vi "TCP - Engine.vi"() -> ()   [LabVIEW 2017]
uses:
  TCP Host/Controls/Read File.ctl
  Controls/RT- Queue States.ctl
  Controls/TCP - Test Settings.ctl
  Controls/TCP - Signal Names.ctl
  Controls/TCP - Signals.ctl
  Controls/TCP - Driver control.ctl
  Variable/SubVI - Global.vi
panel:
  out "Waveform Chart":u32(graph)
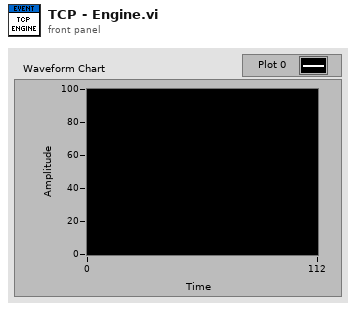
[diagram p1: front panel]
types:
  T1 = typedef "RT- Queue States.ctl" = enum16{"Initialize", "Enqueue", "Enqueue Priority", "Dequeue", "Flush", "Destroy"}
  T2 = typedef "Read File.ctl" = enum16{"Fetch XML", "Open", "Read", "Write", "Close"}
  T3 = typedef "TCP - Driver control.ctl" = enum16{"Init", "Load Sequence File", "Test Running", "Index Step", "Execute Step", "Send Results", "Sequence Complete", "Sequence Aborted", "Stop Sequence Triggered", "Update Manual Values", "Start Aux Logging", "Stop Aux Logging", "Change Dyno Selection", "Reset Emergency Fault", "Get Dyno Config", "Exit"}
  T4 = typedef "TCP - Test Settings.ctl" = cluster{"Sequence File":string, "Iteration":i32}
  T5 = typedef "TCP - Signals.ctl" = cluster{"Signal":T6, "Value":bool, "Data":variant}
  T6 = typedef "TCP - Signal Names.ctl" = enum16{"Test Running", "Start Test", "Test Started", "Sequence Complete", "Seuence Aborted", "Abort Test", "Test Settings Updated", "Log Path", "Update Manual Values", "Start Aux Logging", "Aux Log Started", "Stop Aux Logging", "Aux Log Stopped", "Set Dyno Config", "Get PID Values", "Reset Emergency", "Copy Log File", "Download Files", "Send Test Details", "Generate Alarm"}
  T7 = cluster{"Test details":cluster{"Furnace":string, "Material":string, "Angle":string, "ID":string, "Flowrate":string, "Test Name":string, "Tested By":string}, "Datalog Duration":dbl}
  T8 = cluster{"Furnace":string, "Material":string, "Angle":string, "ID":string, "Flowrate":string, "Test Name":string, "Tested By":string}
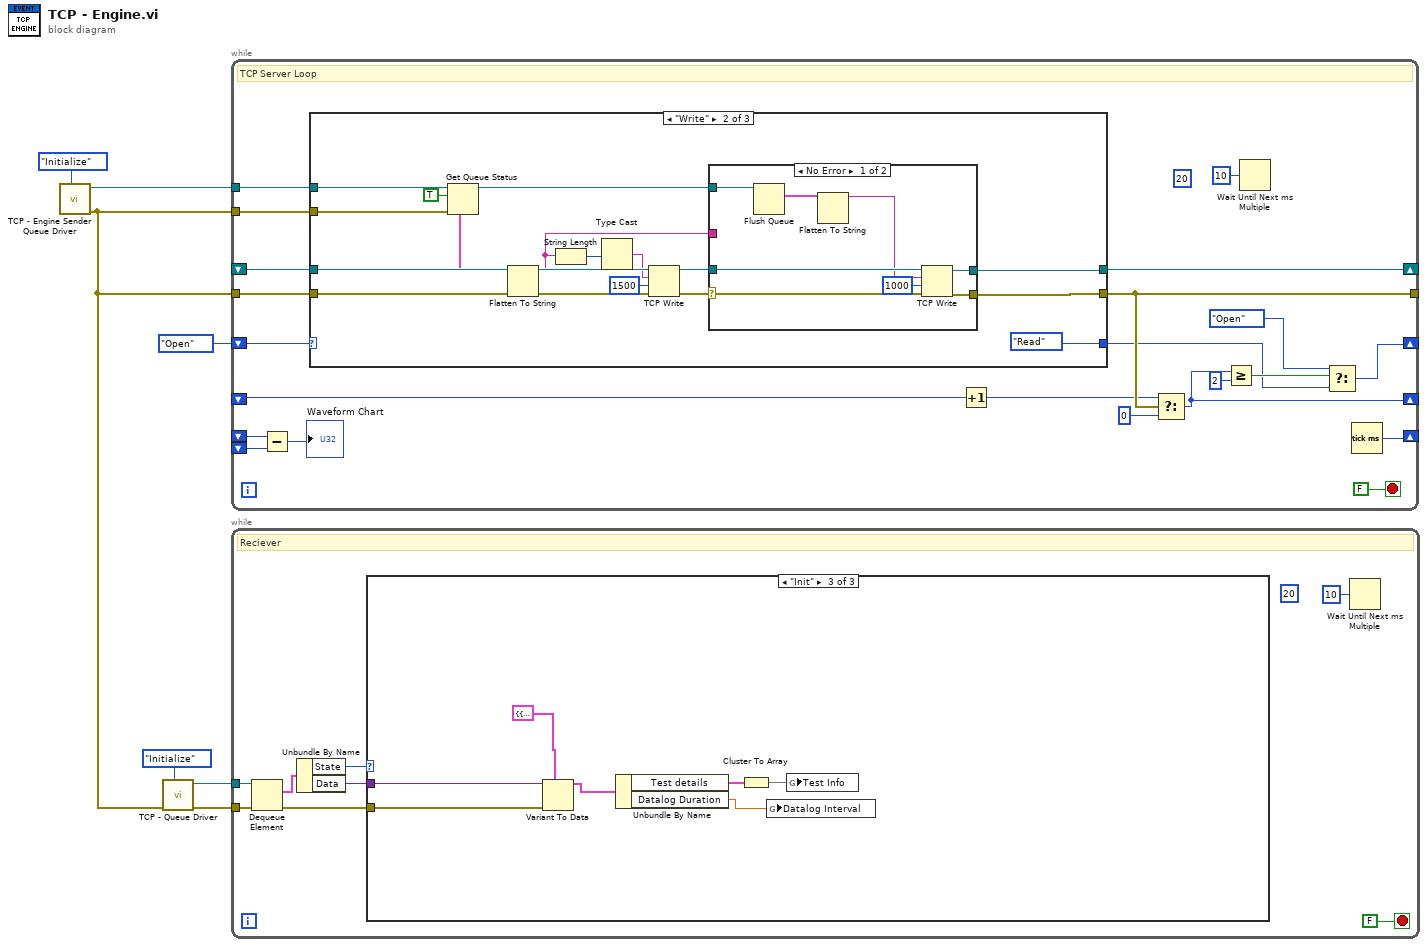
[diagram p0: block diagram]
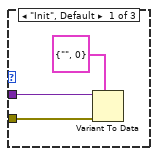
[diagram p2: hidden frame]
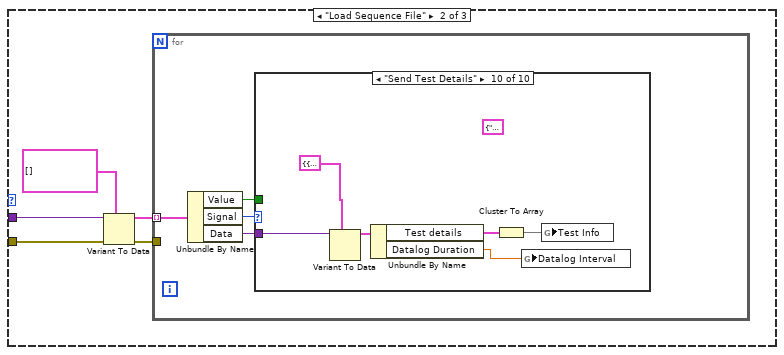
[diagram p3: hidden frame]
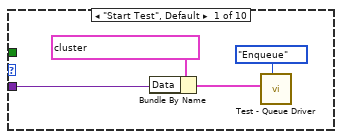
[diagram p4: hidden frame]
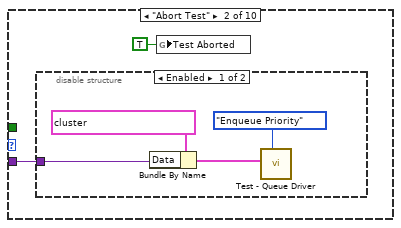
[diagram p5: hidden frame]
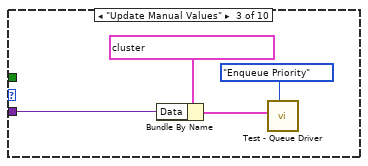
[diagram p7: hidden frame]
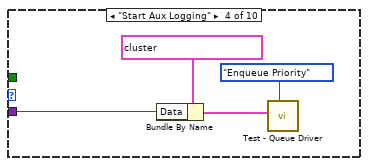
[diagram p8: hidden frame]
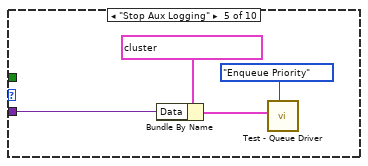
[diagram p9: hidden frame]
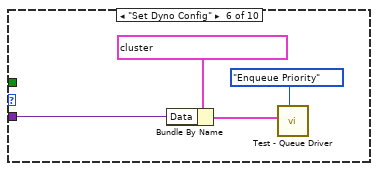
[diagram p10: hidden frame]
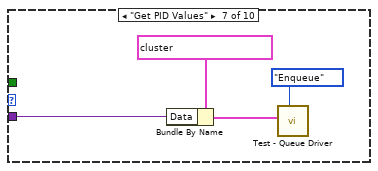
[diagram p11: hidden frame]
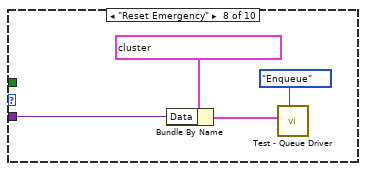
[diagram p12: hidden frame]
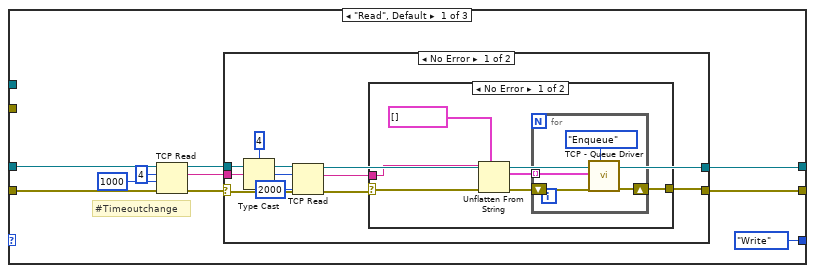
[diagram p14: hidden frame]
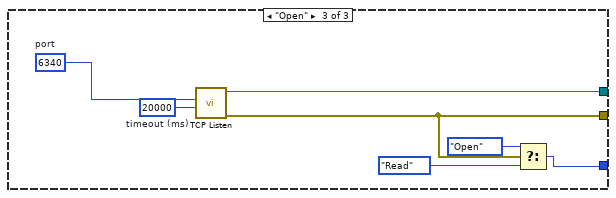
[diagram p18: hidden frame]
diagram:
  n1 = call "TCP - Engine Sender Queue Driver.vi"("Cases"=RT-_Queue_States."Initialize") -> ("error out"=w2:errorcluster, "queue out"=w1:refnum<queue>)  [unwired: 8 in, 1 out]
  n2 = call "TCP - Queue Driver.vi"("Cases"=RT-_Queue_States."Initialize", "error in (no error)"=w2) -> ("error out"=w4:errorcluster, "queue out"=w5:refnum<queue>)  [unwired: 7 in, 1 out]
  n3 = while {
    shift-right: [w28] -> _
    shift-left: _ -> [w27]
    shift-right: [w17] -> _
    shift-left: Read_File."Open" ("R/W") -> [w29]
    shift-right: [w21] -> _
    shift-left: _ -> [w23]
    tunnel: w2 -> [w15]
    tunnel: w1 -> [w14]
    tunnel: w2 -> [w26]
    tunnel: [w25] -> _
    shift-right: [w11] -> _
    shift-left: _ -> [w10]
    shift-left: _ -> [w9]
    stop <- FALSE stop-if-true
    (unwired) u32 20 ("millisecond multiple")
    # "TCP Server Loop"
    n4 = Subtract(x=w10, y=w9) -> (x-y=→"Waveform Chart":u32)
    n5 = case shown="\"Write\"" w29 {
      tunnel: [w34 w76 w95] -> w28
      tunnel: [w33 w75 w94] -> w25
      tunnel: w27 -> [w39 w78 _]
      tunnel: w26 -> [w38 w68 _]
      tunnel: [Read_File."Write" ("R/W") Read_File."Read" ("R/W") w91] -> w13
      tunnel: w15 -> [_ w71 _]
      tunnel: w14 -> [_ w72 _]
      frame "Read", Default {
        # "#Timeoutchange"
        n6 = TCP Read(connection ID=w39, bytes to read=4, error in (no error)=w38, 9:1000 ("timeout ms (25000)")) -> (connection ID out=w37:refnum<k5>, data out=w32:string, error out=w30:errorcluster)  [unwired: 1 out]
        n7 = case shown="No Error" w30 {
          selector: w30 -> [w44 w61]
          tunnel: w37 -> [w49 w62]
          tunnel: [w48 w62] -> w34
          tunnel: [w43 w61] -> w33
          tunnel: w32 -> [w46 _]
          frame No Error {
            n8 = Type Cast(type=4 ("bytes to read"), x=w46) -> (*(type *) &x=w45:i32)
            n9 = TCP Read(connection ID=w49, bytes to read=w45, error in (no error)=w44, 9:2000 ("timeout ms (25000)")) -> (connection ID out=w48:refnum<k5>, data out=w42:string, error out=w41:errorcluster)  [unwired: 1 out]
            n10 = case shown="No Error" w41 {
              selector: w41 -> [w52 w60]
              tunnel: w42 -> [w53 _]
              tunnel: [w55 w60] -> w43
              frame No Error {
                n11 = Unflatten From String(type=cluster{"Data":variant, "State":T3}[] [], binary string=w53, error in (no error)=w52) -> (value=w50:cluster{"Data":variant, "State":T3}[], error out=w51:errorcluster)  [unwired: 2 in, 1 out]
                n12 = for {
                  tunnel: w50 -> [w56] mode=indexing
                  shift-right: [w58] -> w55
                  shift-left: w51 -> [w57]
                  n13 = call "TCP - Queue Driver.vi"("Cases"=RT-_Queue_States."Enqueue", "error in (no error)"=w57, "Element In"=w56) -> ("error out"=w58:errorcluster)  [unwired: 6 in, 2 out]
                }
              }
              frame Error {
              }
            }
          }
          frame Error {
          }
        }
      }
      frame "Write" {
        n14 = Get Queue Status(queue=w72, return elements? (F)=TRUE, error in (no error)=w71) -> (queue out=w63:refnum<queue>, elements=w69:cluster{"Data":variant, "State":T3}[])  [unwired: 6 out]
        n15 = Flatten To String(anything=w69, error in (no error)=w68) -> (data string=w64:string, error out=w67:errorcluster)  [unwired: 2 in, 1 out]
        n16 = String Length(string=w64) -> (length=w66:i32)
        n17 = Type Cast(x=w66) -> (*(type *) &x=w65:string)  [unwired: 1 out]
        n18 = TCP Write(connection ID=w78, data in=w65, error in (no error)=w67, 9:1500 ("timeout ms (25000)")) -> (connection ID out=w77:refnum<k5>, error out=w73:errorcluster)  [unwired: 1 out]
        n19 = case shown="No Error" w73 {
          selector: w73 -> [w84 w88]
          tunnel: w77 -> [w87 w89]
          tunnel: [w86 w89] -> w76
          tunnel: [w85 w88] -> w75
          tunnel: w64 -> [_ _]
          tunnel: w63 -> [w81 _]
          frame No Error {
            n20 = Flush Queue(queue=w81) -> (remaining elements=w82:cluster{"Data":variant, "State":T3}[])  [unwired: 1 in, 2 out]
            n21 = Flatten To String(anything=w82) -> (data string=w80:string)  [unwired: 3 in, 2 out]
            n22 = TCP Write(connection ID=w87, data in=w80, error in (no error)=w84, 9:1000 ("timeout ms (25000)")) -> (connection ID out=w86:refnum<k5>, error out=w85:errorcluster)  [unwired: 1 out]
          }
          frame Error {
          }
        }
      }
      frame "Open" {
        w90 = u16 6340  # port
        w96 = 20000  # timeout (ms)
        n23 = call <vilib>:"TCP Listen.vi"("timeout ms (wait forever: -1)"=w96, "port"=w90) -> ("error out"=w94:errorcluster, "connection ID"=w95:refnum<k5>)  [unwired: 5 in, 3 out]
        n24 = Select(t=Read_File."Open", s=w94, f=Read_File."Read" ("R/W")) -> (s? t:f=w91:T2)
      }
    }
    n25 = Increment(x=w23) -> (x+1=w22:i32)
    n26 = Select(t=w22, s=w25, f=0) -> (s? t:f=w21:i32)
    n27 = Greater Or Equal?(x=w21, y=2) -> (x >= y?=w18:bool)
    n28 = Wait Until Next ms Multiple(millisecond multiple=u32 10) -> ()  [unwired: 1 out]
    n29 = Select(t=Read_File."Open" ("f"), s=w18, f=w13) -> (s? t:f=w17:T2)
    n30 = Tick Count (ms)() -> (millisecond timer value=w11:u32)
  }
  n31 = while {
    tunnel: w5 -> [w103]
    tunnel: w4 -> [w104]
    stop <- FALSE stop-if-true
    (unwired) u32 20 ("millisecond multiple")
    # "Reciever"
    n32 = Dequeue Element(queue=w103, error in (no error)=w104) -> (element=w101:cluster{"Data":variant, "State":T3}, error out=w102:errorcluster)  [unwired: 1 in, 2 out]
    n33 = Unbundle By Name(w101) -> ("State"=w99:T3, "Data"=w98:variant)
    n34 = case shown="\"Send Test Details\"" w99 {
      tunnel: w102 -> [w107 w111 w157]
      tunnel: w98 -> [w106 w112 w158]
      frame "Init", Default {
        n35 = Variant To Data(error in=w107, type=T4 {"Sequence File"="", "Iteration"=0}, Variant=w106) -> ()  [unwired: 2 out]
      }
      frame "Load Sequence File" {
        n36 = Variant To Data(error in=w111, type=T5[] [], Variant=w112) -> (data=w109:T5[], error out=w108:errorcluster)
        n37 = for {
          tunnel: w109 -> [w116] mode=indexing
          tunnel: w108 -> [_]
          n38 = Unbundle By Name(w116) -> ("Value"=w114:bool, "Signal"=w115:T6, "Data"=w113:variant)
          n39 = case shown="\"Send Test Details\"" w115 {
            tunnel: w114 -> [_ _ _ _ _ _ _ _ _ _]
            tunnel: w113 -> [w119 w122 w127 w131 w135 w139 w143 w147 _ w156]
            frame "Start Test", Default {
              n40 = Bundle By Name(cluster=cluster{"Data":variant, "State":T3} {"Data"=variant, "State"=enum."Load Sequence File"} ("Element In"), "Data"=w119) -> (w117:cluster{"Data":variant, "State":T3})
              n41 = call "Test - Queue Driver.vi"("Cases"=RT-_Queue_States."Enqueue", "Element In"=w117) -> ()  [unwired: 7 in, 3 out]
            }
            frame "Abort Test" {
              n42 = disable-structure shown="Enabled" {
                disable-tunnel: w122 -> [w125 _]
                frame Enabled {
                  n43 = Bundle By Name(cluster=cluster{"Data":variant, "State":T3} {"Data"=variant, "State"=enum."Sequence Aborted"} ("Element In"), "Data"=w125) -> (w123:cluster{"Data":variant, "State":T3})
                  n44 = call "Test - Queue Driver.vi"("Cases"=RT-_Queue_States."Enqueue Priority", "Element In"=w123) -> ()  [unwired: 7 in, 3 out]
                }
                frame Disabled {
                }
              }
              n45 = global write "SubVI - Global.vi" "Test Aborted"(TRUE ("Test Aborted")) -> ()
            }
            frame "Update Manual Values" {
              n46 = Bundle By Name(cluster=cluster{"Data":variant, "State":T3} {"Data"=variant, "State"=enum."Update Manual Values"} ("Element In"), "Data"=w127) -> (w128:cluster{"Data":variant, "State":T3})
              n47 = call "Test - Queue Driver.vi"("Cases"=RT-_Queue_States."Enqueue Priority", "Element In"=w128) -> ()  [unwired: 7 in, 3 out]
            }
            frame "Start Aux Logging" {
              n48 = Bundle By Name(cluster=cluster{"Data":variant, "State":T3} {"Data"=variant, "State"=enum."Start Aux Logging"} ("Element In"), "Data"=w131) -> (w132:cluster{"Data":variant, "State":T3})
              n49 = call "Test - Queue Driver.vi"("Cases"=RT-_Queue_States."Enqueue Priority", "Element In"=w132) -> ()  [unwired: 7 in, 3 out]
            }
            frame "Stop Aux Logging" {
              n50 = Bundle By Name(cluster=cluster{"Data":variant, "State":T3} {"Data"=variant, "State"=enum."Stop Aux Logging"} ("Element In"), "Data"=w135) -> (w136:cluster{"Data":variant, "State":T3})
              n51 = call "Test - Queue Driver.vi"("Cases"=RT-_Queue_States."Enqueue Priority", "Element In"=w136) -> ()  [unwired: 7 in, 3 out]
            }
            frame "Set Dyno Config" {
              n52 = Bundle By Name(cluster=cluster{"Data":variant, "State":T3} {"Data"=variant, "State"=enum."Change Dyno Selection"} ("Element In"), "Data"=w139) -> (w140:cluster{"Data":variant, "State":T3})
              n53 = call "Test - Queue Driver.vi"("Cases"=RT-_Queue_States."Enqueue Priority", "Element In"=w140) -> ()  [unwired: 7 in, 3 out]
            }
            frame "Get PID Values" {
              n54 = Bundle By Name(cluster=cluster{"Data":variant, "State":T3} {"Data"=variant, "State"=enum."Get Dyno Config"} ("Element In"), "Data"=w143) -> (w144:cluster{"Data":variant, "State":T3})
              n55 = call "Test - Queue Driver.vi"("Cases"=RT-_Queue_States."Enqueue", "Element In"=w144) -> ()  [unwired: 7 in, 3 out]
            }
            frame "Reset Emergency" {
              n56 = Bundle By Name(cluster=cluster{"Data":variant, "State":T3} {"Data"=variant, "State"=enum."Reset Emergency Fault"} ("Element In"), "Data"=w147) -> (w148:cluster{"Data":variant, "State":T3})
              n57 = call "Test - Queue Driver.vi"("Cases"=RT-_Queue_States."Enqueue", "Element In"=w148) -> ()  [unwired: 7 in, 3 out]
            }
            frame "Download Files" {
            }
            frame "Send Test Details" {
              (unwired) T8 {"Furnace"="Furnace A", "Material"="Coke", "Angle"="Multi Angle", "ID"="Trajectory 9", "Flowrate"="Flow", "Test Name"="Coke Burn", "Tested By"="Anirban"} ("Test details")
              n58 = Variant To Data(type=T7 {"Test details"={"Furnace"="Furnace A", "Material"="Aluminium", "Angle"="Multi Angle", "ID"="Trajectory 9", "Flowrate"="Flow", "Test Name"="Coke Burn", "Tested By"="Anirban"}, "Datalog Duration"=0.0}, Variant=w156) -> (data=w153:T7)  [unwired: 1 in, 1 out]
              n59 = Unbundle By Name(w153) -> ("Test details"=w152:T8, "Datalog Duration"=w151:dbl)
              n60 = Cluster To Array(cluster=w152) -> (array=w155:string[])
              n61 = global write "SubVI - Global.vi" "Datalog Interval"(w151) -> ()
              n62 = global write "SubVI - Global.vi" "Test Info"(w155) -> ()
            }
          }
        }
      }
      frame "Init" {
        n63 = Variant To Data(error in=w157, type=T7 {"Test details"={"Furnace"="Furnace A", "Material"="Aluminium", "Angle"="Multi Angle", "ID"="Trajectory 9", "Flowrate"="Flow", "Test Name"="Coke Burn", "Tested By"="Anirban"}, "Datalog Duration"=0.0}, Variant=w158) -> (data=w161:T7)  [unwired: 1 out]
        n64 = Unbundle By Name(w161) -> ("Test details"=w160:T8, "Datalog Duration"=w159:dbl)
        n65 = Cluster To Array(cluster=w160) -> (array=w163:string[])
        n66 = global write "SubVI - Global.vi" "Datalog Interval"(w159) -> ()
        n67 = global write "SubVI - Global.vi" "Test Info"(w163) -> ()
      }
    }
    n68 = Wait Until Next ms Multiple(millisecond multiple=u32 10) -> ()  [unwired: 1 out]
  }
